vi "GDSLvIcon_ResizeTextIcon.vi"(1 "IconIn":u8[][](array[numeric]) format="%x", 2 "Rows/Height":u8, 3 "Columns/Width":i32, 5 "error in (no error)":errorcluster) -> (15 "IconOut":u8[][](array[numeric]) format="%x", 19 "error out":errorcluster)   [LabVIEW 2012]
uses:
  <vilib>/Analysis/NI_AALBase.lvlib
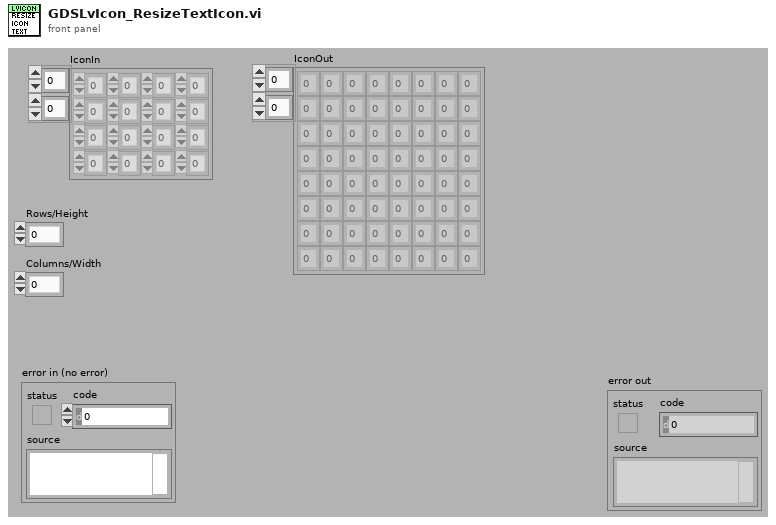
[diagram p1: front panel]
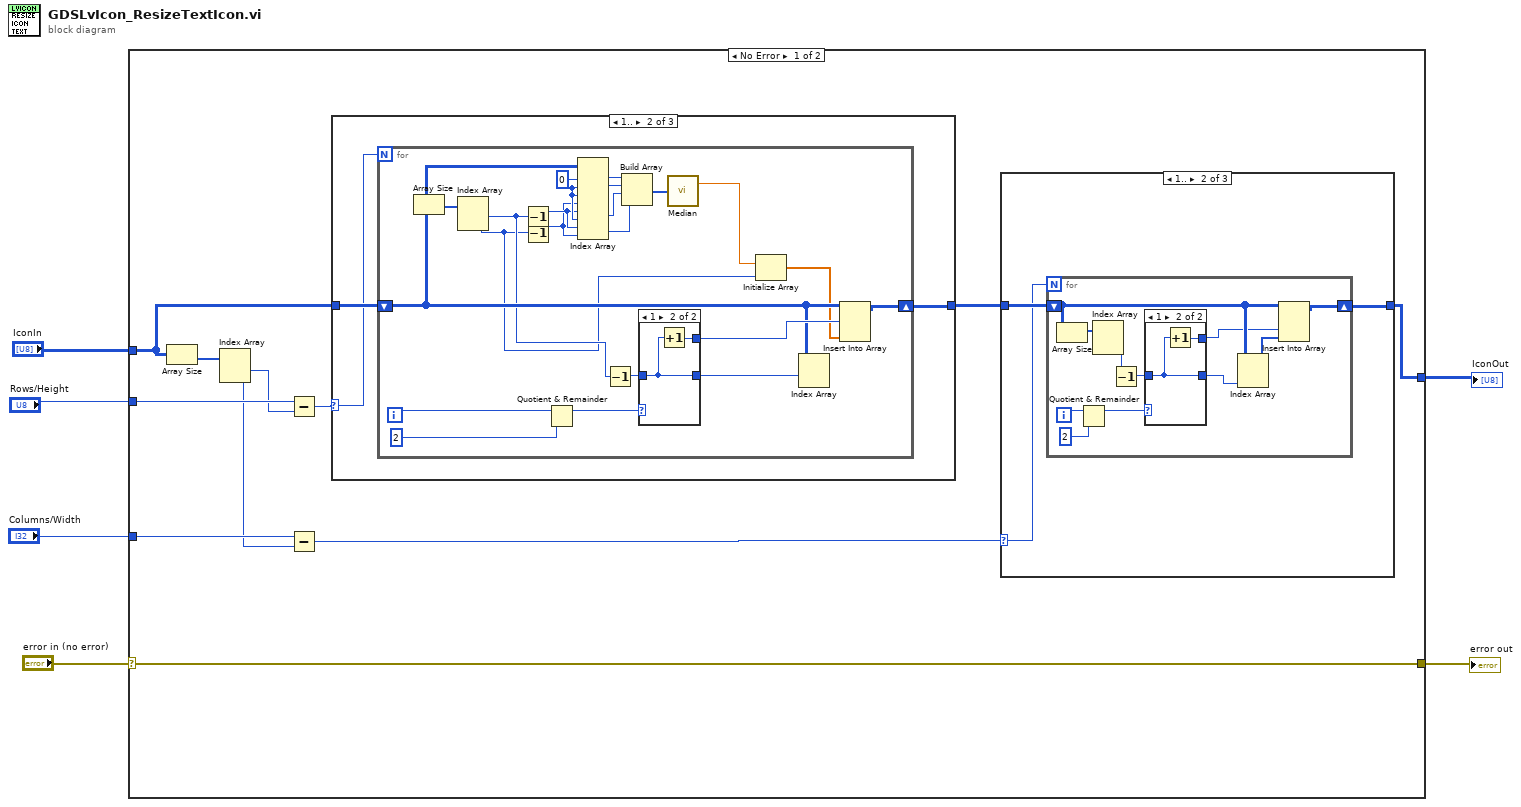
[diagram p0: block diagram]
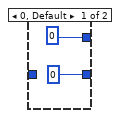
[diagram p3: hidden frame]
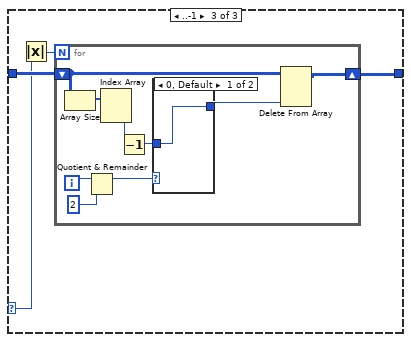
[diagram p4: hidden frame]
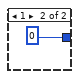
[diagram p5: hidden frame]
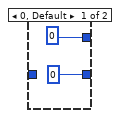
[diagram p7: hidden frame]
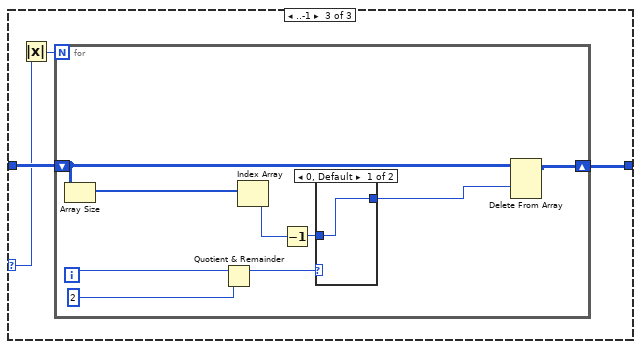
[diagram p8: hidden frame]
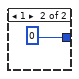
[diagram p9: hidden frame]
diagram:
  n1 = case shown="No Error" "error in (no error)" {
    selector: "error in (no error)" -> [w17 w97]
    tunnel: [w17 w97] -> w5
    tunnel: "IconIn" -> [w13 w96]
    tunnel: [w12 w96] -> w3
    tunnel: "Rows/Height" -> [w15 _]
    tunnel: "Columns/Width" -> [w10 _]
    frame No Error {
      n2 = Array Size(array=w13) -> (size(s)=w16:i32[])
      n3 = Index Array(array=w16) -> (element #1=w9:i32, element #2=w7:i32)  [unwired: 2 in]
      n4 = Subtract(x=w15, y=w9) -> (x-y=w14:i32)
      n5 = Subtract(x=w10, y=w7) -> (x-y=w8:i32)
      n6 = case shown="1.." w14 {
        selector: w14 -> [_ w54 w83]
        tunnel: w13 -> [w52 w55 w84]
        tunnel: [w52 w53 w82] -> w11
        frame 0, Default {
        }
        frame 1.. {
          n7 = for {
            N: w54 -> [_]
            shift-right: [w73] -> w53
            shift-left: w55 -> [w60]
            i -> [w76]
            w68 = 0 ("index (row)")
            n8 = Array Size(array=w60) -> (size(s)=w69:i32[])
            n9 = Index Array(array=w69) -> (element #1=w59:i32, element #2=w58:i32)  [unwired: 2 in]
            n10 = Decrement(x=w59) -> (x-1=w67:i32)
            n11 = Decrement(x=w58) -> (x-1=w66:i32)
            n12 = Quotient & Remainder(x=w76, y=2) -> (x-y*floor(x/y)=w71:i32)  [unwired: 1 out]
            n13 = Index Array(array=w60, index (row) #1=w68, index (col) #1=w68, index (row) #2=w68, index (col) #2=w66, index (row) #3=w67, index (col) #3=w68, index (row) #4=w67, index (col) #4=w66) -> (element #1=w65:u8, element #2=w64:u8, element #3=w63:u8, element #4=w62:u8)
            n14 = Decrement(x=w59) -> (x-1=w70:i32)
            n15 = Build Array(w65, w64, w63, w62) -> (w61:u8[])
            n16 = case shown="1" w71 {
              tunnel: [0 ("index (row)") w79] -> w74
              tunnel: [0 ("index (row)") w80] -> w72
              tunnel: w70 -> [_ w79]
              frame 0, Default {
              }
              frame 1 {
                n17 = Increment(x=w79) -> (x+1=w80:i32)
              }
            }
            n18 = call <vilib>:"Median.vi"("X"=w61) -> ("median"=w57:dbl)  [unwired: 1 out]
            n19 = Initialize Array(w57, w58) -> (w56:dbl[])
            n20 = Index Array(array=w60, index (row)=w74) -> ()  [unwired: 1 in, 1 out]
            n21 = Insert Into Array(array=w60, index (row)=w72, new element=w56) -> (w73:u8[][])  [unwired: 1 in]
          }
        }
        frame ..-1 {
          n22 = Absolute Value(x=w83) -> (abs(x)=w81:i32)
          n23 = for {
            N: w81 -> [_]
            shift-right: [w86] -> w82
            shift-left: w84 -> [w87]
            i -> [w93]
            n24 = Array Size(array=w87) -> (size(s)=w90:i32[])
            n25 = Quotient & Remainder(x=w93, y=2) -> (x-y*floor(x/y)=w91:i32)  [unwired: 1 out]
            n26 = Index Array(array=w90) -> (element=w89:i32)  [unwired: 1 in]
            n27 = Decrement(x=w89) -> (x-1=w88:i32)
            n28 = case shown="0, Default" w91 {
              tunnel: [w94 0 ("index (row)")] -> w85
              tunnel: w88 -> [w94 _]
              frame 0, Default {
              }
              frame 1 {
              }
            }
            n29 = Delete From Array(array=w87, index (row)=w85) -> (array with subset deleted=w86:u8[][])  [unwired: 2 in, 1 out]
          }
        }
      }
      n30 = case shown="1.." w8 {
        selector: w8 -> [_ w20 w39]
        tunnel: w11 -> [w18 w21 w40]
        tunnel: [w18 w19 w38] -> w12
        frame 0, Default {
        }
        frame 1.. {
          n31 = for {
            N: w20 -> [_]
            shift-right: [w29] -> w19
            shift-left: w21 -> [w27]
            i -> [w32]
            n32 = Array Size(array=w27) -> (size(s)=w26:i32[])
            n33 = Quotient & Remainder(x=w32, y=2) -> (x-y*floor(x/y)=w28:i32)  [unwired: 1 out]
            n34 = Index Array(array=w26) -> (element #2=w24:i32)  [unwired: 2 in, 1 out]
            n35 = Decrement(x=w24) -> (x-1=w25:i32)
            n36 = case shown="1" w28 {
              tunnel: [0 ("index (row)") w35] -> w22
              tunnel: [0 ("index (row)") w36] -> w23
              tunnel: w25 -> [_ w35]
              frame 0, Default {
              }
              frame 1 {
                n37 = Increment(x=w35) -> (x+1=w36:i32)
              }
            }
            n38 = Index Array(array=w27, index (col)=w22) -> (element=w30:u8[])  [unwired: 1 in]
            n39 = Insert Into Array(array=w27, index (col)=w23, new element=w30) -> (w29:u8[][])  [unwired: 1 in]
          }
        }
        frame ..-1 {
          n40 = Absolute Value(x=w39) -> (abs(x)=w37:i32)
          n41 = for {
            N: w37 -> [_]
            shift-right: [w43] -> w38
            shift-left: w40 -> [w44]
            i -> [w49]
            n42 = Array Size(array=w44) -> (size(s)=w46:i32[])
            n43 = Quotient & Remainder(x=w49, y=2) -> (x-y*floor(x/y)=w47:i32)  [unwired: 1 out]
            n44 = Index Array(array=w46) -> (element #2=w42:i32)  [unwired: 2 in, 1 out]
            n45 = Decrement(x=w42) -> (x-1=w45:i32)
            n46 = case shown="0, Default" w47 {
              tunnel: [w50 0 ("index (row)")] -> w41
              tunnel: w45 -> [w50 _]
              frame 0, Default {
              }
              frame 1 {
              }
            }
            n47 = Delete From Array(array=w44, index (col)=w41) -> (array with subset deleted=w43:u8[][])  [unwired: 2 in, 1 out]
          }
        }
      }
    }
    frame Error {
    }
  }
  "error out" <- w5
  "IconOut" <- w3
